vi "dfd_Classical IIR Filter Design Params Validation.vi"(4 "params":dbl[](array[numeric]) format="%.2f", 6 "fs [Hz]":dbl=1.0 format="%.2f", 7 "filter type":T1(ring), 8 "error in (no error)":errorcluster, 9 "low cutoff freq: fl":dbl, 10 "high cutoff freq: fh":dbl, 11 "order":i32) -> (0 "error out":errorcluster)   [LabVIEW 2017, in "NI_DigFilterLicensed.lvlib"]
uses:
  <vilib>/addons/Digital Filter Design/NI_DigFilterLicensed.lvlib
  <vilib>/addons/Digital Filter Design/_Misc.llb/dfd_Error Handlers (Multiple).vi
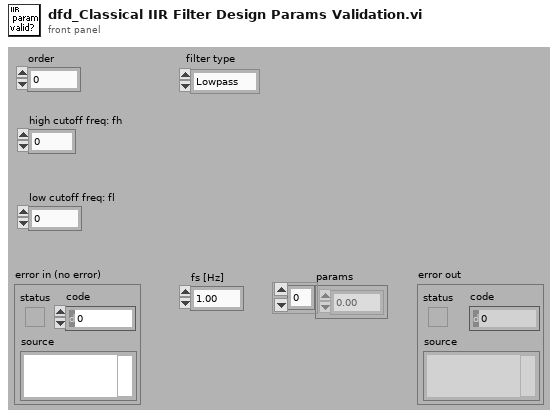
[diagram p1: front panel]
types:
  T1 = enum16{"Lowpass", "Highpass", "Bandpass", "Bandstop"}
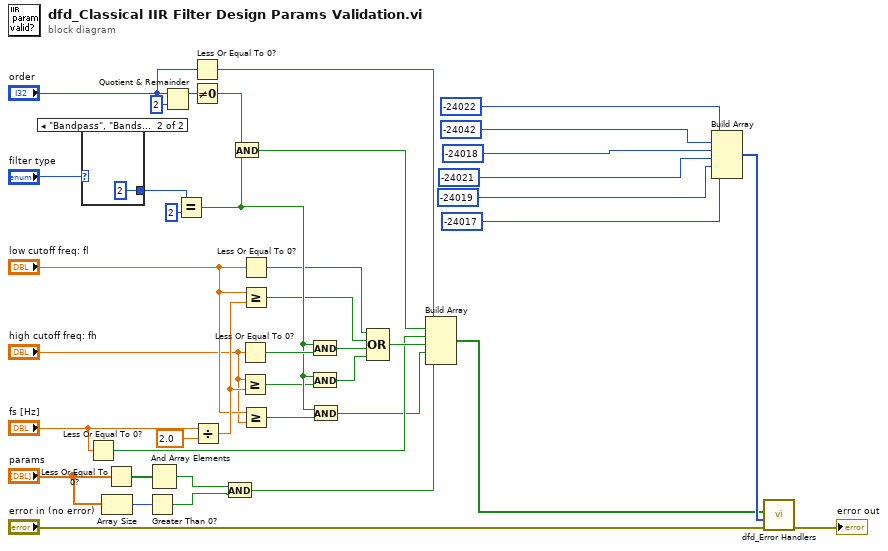
[diagram p0: block diagram]
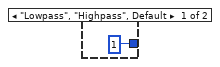
[diagram p2: hidden frame]
diagram:
  n1 = case shown="\"Bandpass\", \"Bandstop\"" "filter type" {
    tunnel: [1 2] -> w40
    frame "Lowpass", "Highpass", Default {
    }
    frame "Bandpass", "Bandstop" {
    }
  }
  n2 = Less Or Equal To 0?(x="fs [Hz]") -> (x <= 0?=w2:bool)
  n3 = Array Size(array="params") -> (size(s)=w19:i32)
  n4 = Less Or Equal To 0?(x="params") -> (x <= 0?=w32:bool[])
  n5 = Greater Than 0?(x=w19) -> (x > 0?=w16:bool)
  n6 = And Array Elements(Boolean array=w32) -> (logical AND=w17:bool)
  n7 = Quotient & Remainder(x="order", y=2) -> (x-y*floor(x/y)=w34:i32)  [unwired: 1 out]
  n8 = Equal?(x=w40, y=2) -> (x = y?=w9:bool)
  n9 = Less Or Equal To 0?(x="order") -> (x <= 0?=w28:bool)
  n10 = Not Equal To 0?(x=w34) -> (x != 0?=w30:bool)
  n11 = Divide(x="fs [Hz]", y=2.0) -> (x/y=w15:dbl)
  n12 = And(x=w17, y=w16) -> (x .and. y?=w18:bool)
  n13 = And(x=w30, y=w9) -> (x .and. y?=w29:bool)
  n14 = Less Or Equal To 0?(x="high cutoff freq: fh") -> (x <= 0?=w10:bool)
  n15 = Greater Or Equal?(x="high cutoff freq: fh", y=w15) -> (x >= y?=w8:bool)
  n16 = Less Or Equal To 0?(x="low cutoff freq: fl") -> (x <= 0?=w5:bool)
  n17 = Greater Or Equal?(x="low cutoff freq: fl", y=w15) -> (x >= y?=w6:bool)
  n18 = Greater Or Equal?(x="low cutoff freq: fl", y="high cutoff freq: fh") -> (x >= y?=w22:bool)
  n19 = And(x=w9, y=w10) -> (x .and. y?=w7:bool)
  n20 = And(x=w9, y=w8) -> (x .and. y?=w12:bool)
  n21 = And(x=w9, y=w22) -> (x .and. y?=w1:bool)
  n22 = Compound Arithmetic op=OR(w5, w6, w7, w12) -> (w13:bool)
  n23 = Build Array(w28, w29, w2, w13, w1, w18) -> (w23:bool[])
  n24 = Build Array(-24022 ("ERR_ORDER_LE_ZERO"), -24042 ("ERR_CLASSICAL_IIR_BP_BS_ORDER"), -24018 ("ERR_FS_LE_ZERO"), -24021 ("ERR_FREQ_RANGE_WRONG"), -24019 ("ERR_FREQ_NOT_ASCENDING"), -24017 ("ERR_dB_LE_ZERO")) -> (w24:i32[])
  n25 = call-poly <vilib>:"dfd_Error Handlers.vi"("error in (no error)"="error in (no error)", "error sources"=w24, "condition failed?"=w23) -> ("error out"=→"error out":errorcluster)  [unwired: 8 out]
